vi "hysteresisLiveCompObjectiveFunction.vi"(3 "output control":T1, 4 "data":variant, 5 "X":dbl[](array[numeric])) -> (0 "error out":errorcluster, 1 "gradient":dbl[](array[numeric]), 2 "f(X)":dbl)   [LabVIEW 2016]
doc: "This template is the starting point for creating an objectivel function to be passed to the Unconstrained Optimization.vi."
panel:
  out "distoredDataOut":dbl[][](graph)
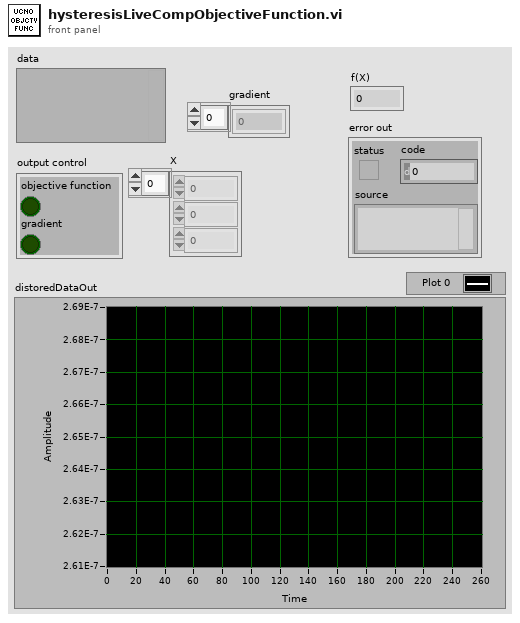
[diagram p1: front panel]
types:
  T1 = cluster{"objective function":bool, "gradient":bool}
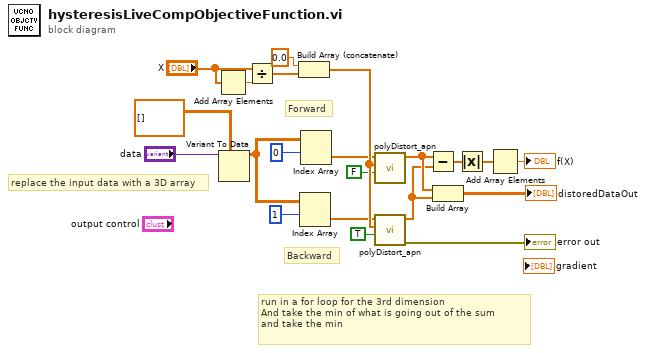
[diagram p0: block diagram]
diagram:
  # "Backward"
  # "Forward"
  # "run in a for loop for the 3rd dimension\nAnd take the min of what is going out of the sum\nand take the min"
  # "replace the input data with a 3D array"
  n1 = Add Array Elements(numeric array="X") -> (sum=w11:dbl)
  n2 = Variant To Data(type=dbl[][] [], Variant="data") -> (data=w19:dbl[][])  [unwired: 1 in, 1 out]
  n3 = Divide(x="X", y=w11) -> (x/y=w13:dbl[])
  n4 = Build Array (concatenate)(0.0, w13) -> (w17:dbl[])
  n5 = Index Array(array=w19, index (row)=1 ("disabled index (col)")) -> (element=w6:dbl[])  [unwired: 1 in]
  n6 = Index Array(array=w19, index (row)=0) -> (element=w7:dbl[])  [unwired: 1 in]
  n7 = call "polyDistort_apn.vi"("Backward?"=FALSE, "polyIn"=w17, "lineDataIn"=w7) -> ("distoredDataOut"=w16:dbl[])  [unwired: 7 in, 1 out]
  n8 = call "polyDistort_apn.vi"("Backward?"=TRUE, "polyIn"=w17, "lineDataIn"=w6) -> ("error out"=→"error out":errorcluster, "distoredDataOut"=w15:dbl[])  [unwired: 7 in]
  n9 = Subtract(x=w16, y=w15) -> (x-y=w10:dbl[])
  n10 = Build Array(w16, w15) -> (→"distoredDataOut":dbl[][])
  n11 = Absolute Value(x=w10) -> (abs(x)=w5:dbl[])
  n12 = Add Array Elements(numeric array=w5) -> (sum=→"f(X)":dbl)
